vi "Global_CMD.vi"() -> ()   [LabVIEW 2017, in "Rotation_Overloard.lvlib"]
uses:
  Rotation_Overloard.lvlib
  CLUSTER_Rotation_CMD.ctl
  ENUM_Rotation_Positon.ctl
panel:
  in  "CMD_SM_Rotation":T1={"Rotation Positon"=enum."Neutral", "Enable Rotation"=TRUE}
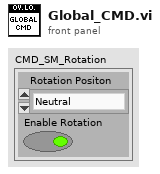
[diagram p1: front panel]
types:
  T1 = typedef "Rotation_Overloard.lvlib/CLUSTER_Rotation_CMD.ctl" = cluster{"Rotation Positon":T2, "Enable Rotation":bool}
  T2 = typedef "Rotation_Overloard.lvlib/ENUM_Rotation_Positon.ctl" = enum16{"Neutral", "Pickup", "Exchange", "Switch", "Scale", "Climb", "Manual"}
diagram:
